vi "ZeroPos.vi"(0 "object in":refnum<class "Prior_Zmotor.lvclass">, 5 "error in (no error)":errorcluster) -> (14 "object out":refnum<class "Prior_Zmotor.lvclass">, 19 "error out":errorcluster)   [LabVIEW 2021, in "Prior_Zmotor.lvclass"]
uses:
  Prior_Zmotor.lvclass
  Prior_Zmotor.lvclass/Prior_Zmotor.ctl
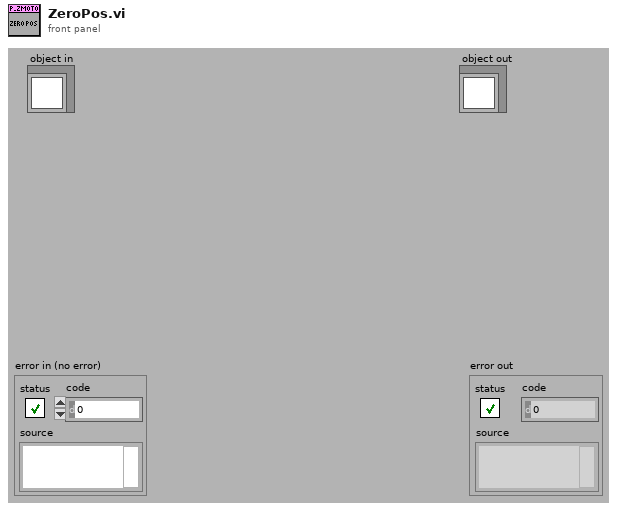
[diagram p1: front panel]
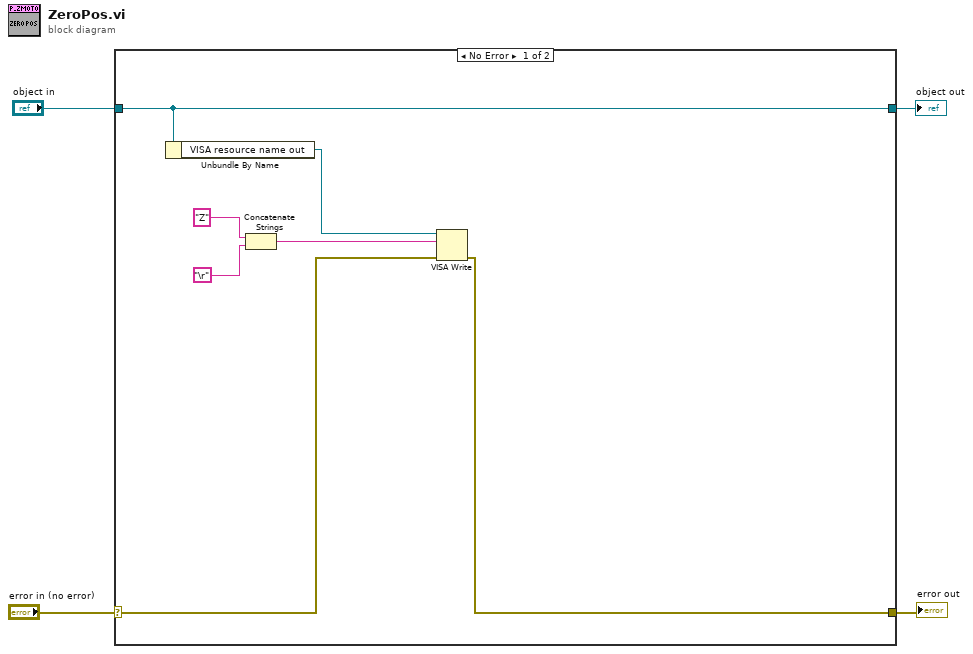
[diagram p0: block diagram]
diagram:
  n1 = case shown="No Error" "error in (no error)" {
    selector: "error in (no error)" -> [w9 w13]
    tunnel: [w8 w13] -> w3
    tunnel: [w11 w12] -> w1
    tunnel: "object in" -> [w11 w12]
    frame No Error {
      n2 = Unbundle By Name(w11) -> ("VISA resource name out"=w10:refnum<visa-resource-name>)
      n3 = Concatenate Strings("Z" ("write buffer"), "\r") -> (w5:string)
      n4 = VISA Write(VISA resource name=w10, write buffer=w5, error in (no error)=w9) -> (error out=w8:errorcluster)  [unwired: 2 out]
    }
    frame Error {
    }
  }
  "error out" <- w3
  "object out" <- w1
